vi "ReadBGorCali (SubVI) - Copy.vi"(7 "DataType":enum16{"BG", "Cali"}(ring), 8 "error in (no error)":errorcluster, 11 "file path in":path) -> (0 "error out":errorcluster, 2 "CtrlVCluster":T1, 3 "AvgDataCluster":T2)   [LabVIEW 2020]
panel:
  out "Waveform Graph":dbl[][](graph)
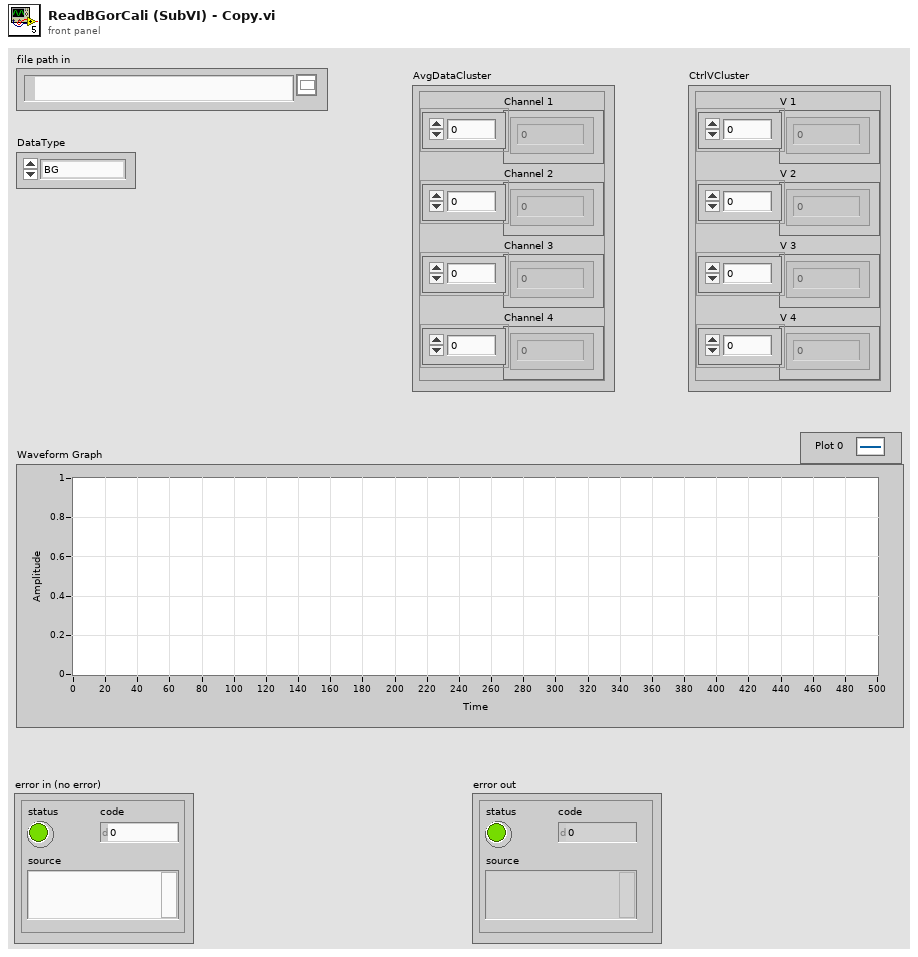
[diagram p1: front panel]
types:
  T1 = cluster{"V 1":dbl[], "V 2":dbl[], "V 3":dbl[], "V 4":dbl[]}
  T2 = cluster{"Channel 1":dbl[], "Channel 2":dbl[], "Channel 3":dbl[], "Channel 4":dbl[]}
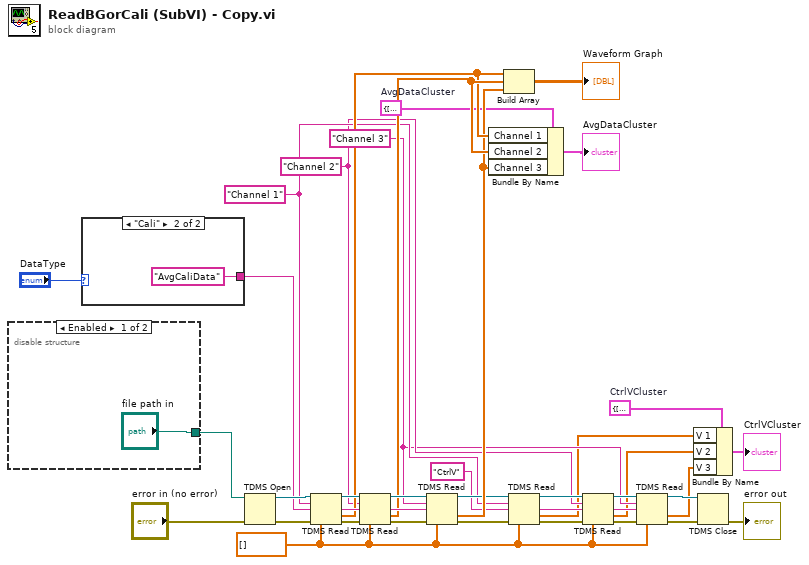
[diagram p0: block diagram]
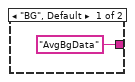
[diagram p2: hidden frame]
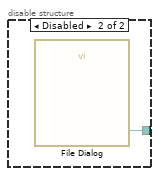
[diagram p3: hidden frame]
diagram:
  w1 = T2 {"Channel 1"=[], "Channel 2"=[], "Channel 3"=[], "Channel 4"=[]}  # AvgDataCluster
  w3 = T1 {"V 1"=[], "V 2"=[], "V 3"=[], "V 4"=[]}  # CtrlVCluster
  w12 = "Channel 3" ("group name in")
  w13 = "Channel 2" ("group name in")
  w11 = dbl[] []
  w16 = "Channel 1" ("group name in")
  n1 = disable-structure shown="Enabled" {
    disable-tunnel: ["file path in" w41] -> w36
    frame Enabled {
    }
    frame Disabled {
      n2 = call "File Dialog"() -> ("selected path"=w41:path)  [unwired: 12 in, 3 out]
    }
  }
  n3 = case shown="\"Cali\"" "DataType" {
    tunnel: ["AvgBgData" "AvgCaliData"] -> w4
    frame "BG", Default {
    }
    frame "Cali" {
    }
  }
  n4 = TDMS Open(8:"error in (no error)", 11:w36) -> (0:w38:errorcluster, 3:w39:refnum<k34>)  [unwired: 5 in]
  n5 = TDMS Read(0:w39, 5:w16, 7:w4, 11:w38, 12:w11) -> (4:w35:refnum<k34>, 8:w33:string, 10:w26:dbl[], 15:w34:errorcluster)  [unwired: 3 in, 2 out]
  n6 = TDMS Read(0:w35, 5:w13, 7:w33, 11:w34, 12:w11) -> (4:w32:refnum<k34>, 8:w30:string, 10:w28:dbl[], 15:w31:errorcluster)  [unwired: 3 in, 2 out]
  n7 = TDMS Read(0:w32, 5:w12, 7:w30, 11:w31, 12:w11) -> (4:w24:refnum<k34>, 10:w25:dbl[], 15:w20:errorcluster)  [unwired: 3 in, 3 out]
  n8 = Bundle By Name(cluster=w1, "Channel 1"=w26, "Channel 2"=w28, "Channel 3"=w25) -> (→"AvgDataCluster":T2)
  n9 = Build Array(w26, w28, w25) -> (→"Waveform Graph":dbl[][])
  n10 = TDMS Read(0:w24, 5:w16, 7:"CtrlV" ("group name in"), 11:w20, 12:w11) -> (4:w23:refnum<k34>, 8:w15:string, 10:w10:dbl[], 15:w19:errorcluster)  [unwired: 3 in, 2 out]
  n11 = TDMS Read(0:w23, 5:w13, 7:w15, 11:w19, 12:w11) -> (4:w22:refnum<k34>, 8:w14:string, 10:w9:dbl[], 15:w18:errorcluster)  [unwired: 3 in, 2 out]
  n12 = TDMS Read(0:w22, 5:w12, 7:w14, 11:w18, 12:w11) -> (4:w21:refnum<k34>, 10:w8:dbl[], 15:w6:errorcluster)  [unwired: 3 in, 3 out]
  n13 = Bundle By Name(cluster=w3, "V 1"=w10, "V 2"=w9, "V 3"=w8) -> (→"CtrlVCluster":T1)
  n14 = TDMS Close(8:w6, 11:w21) -> (0:→"error out":errorcluster)  [unwired: 1 out]
